vi "Analisi.vi"(6 "Cluster COLORS":cluster{"fore":u32, "back ER":u32, "back":u32}={"fore"=10197915, "back ER"=11796480, "back"=43}, 7 "crea\ntabella scarti":bool, 8 "MCListbox tabella dati":refnum<vi>, 9 "n colonna":i32, 10 "Array index eliminati in":i32[](array[numeric]), 11 "Array":string[](array[string])) -> (2 "Array index eliminati":i32[](array[numeric]))   [LabVIEW 2016]
uses:
  formule.llb/PASSI.ctl
  formule.llb/Global.vi
panel:
  in  "start index (0)":i32
  out "index of element":i32
  out "element":string
  in  "eliminati":i32
  out "Array 2":string[](array[string])
  in  "index":i32
  in  "PASSO":T1
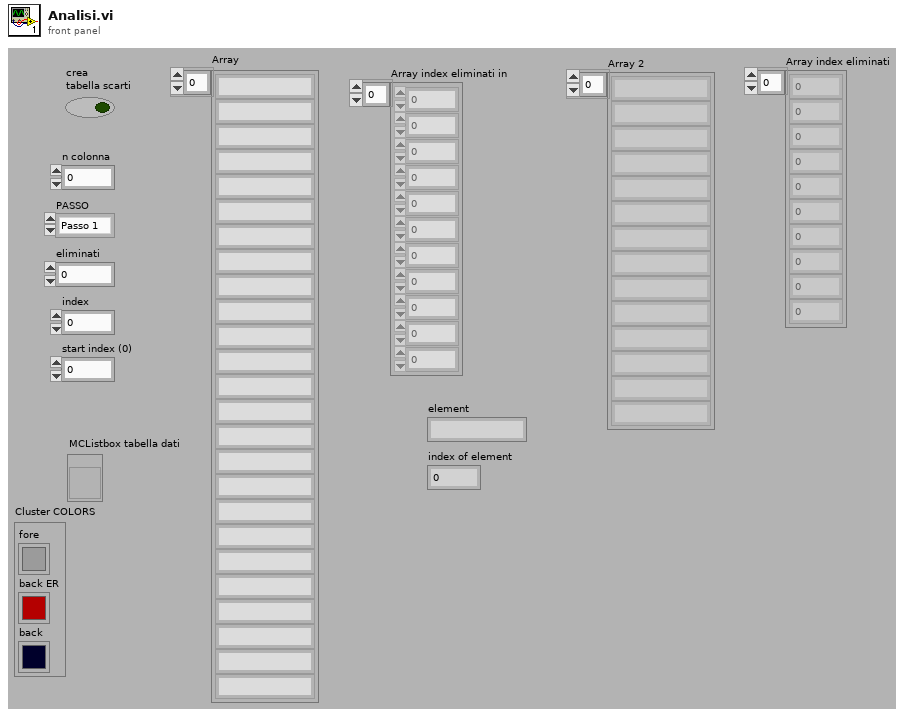
[diagram p1: front panel]
types:
  T1 = typedef "PASSI.ctl" = enum16{"Passo 1", "Passo 2", "Passo 3", "Passo 4", "Passo 5"}
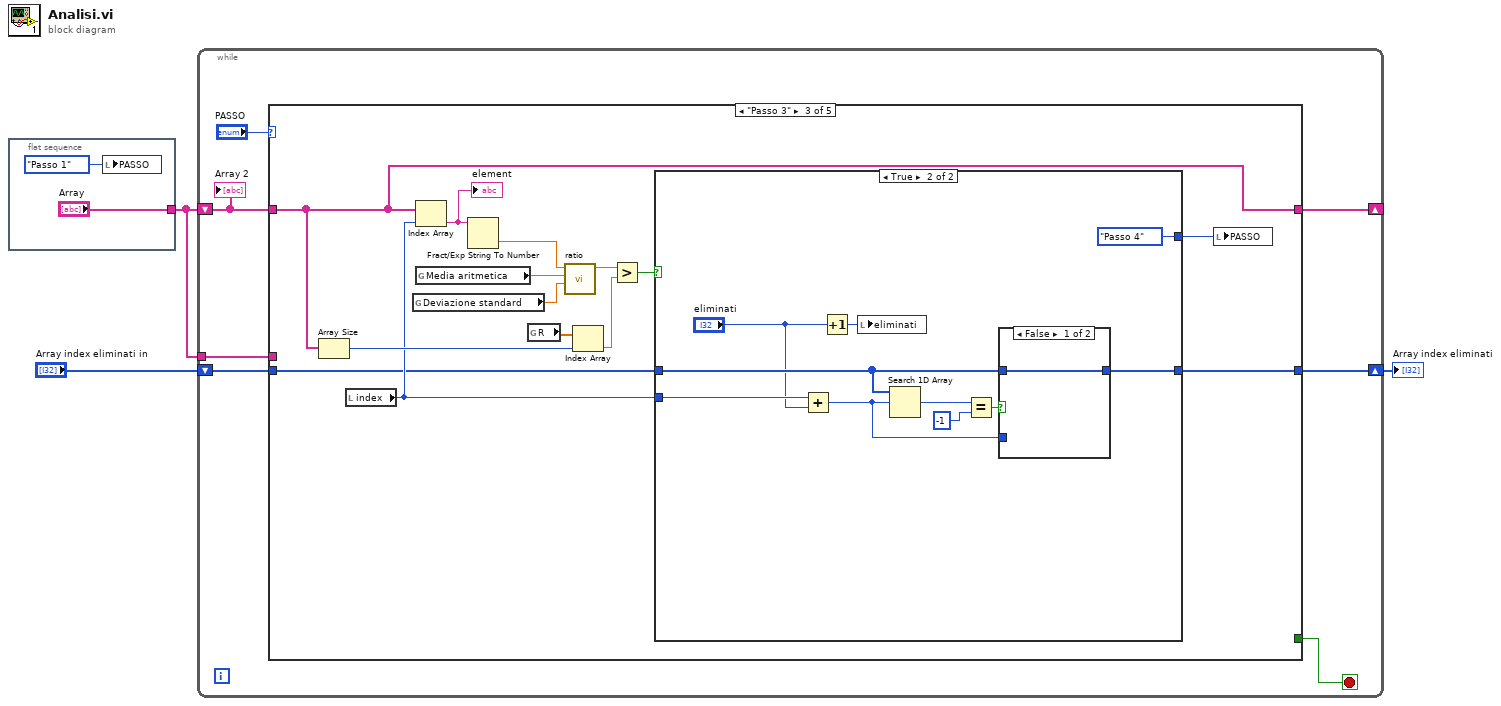
[diagram p0: block diagram]
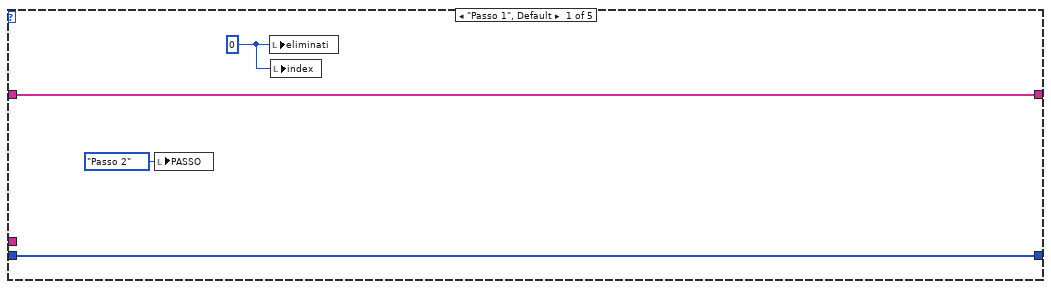
[diagram p2: hidden frame]
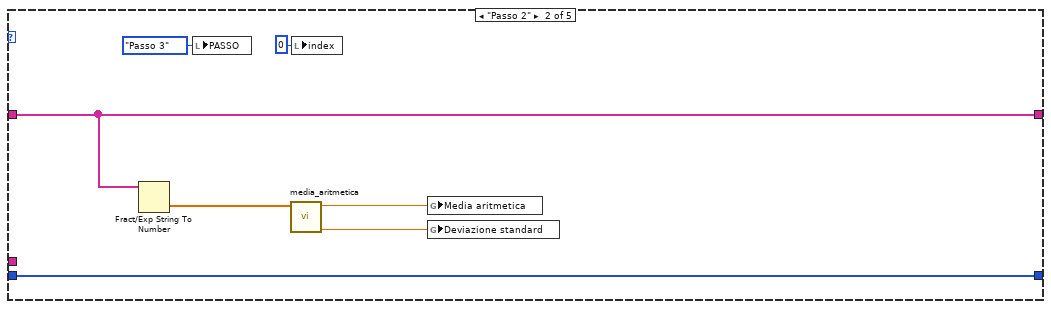
[diagram p3: hidden frame]
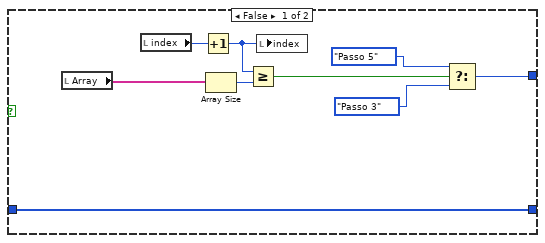
[diagram p4: hidden frame]
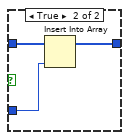
[diagram p5: hidden frame]
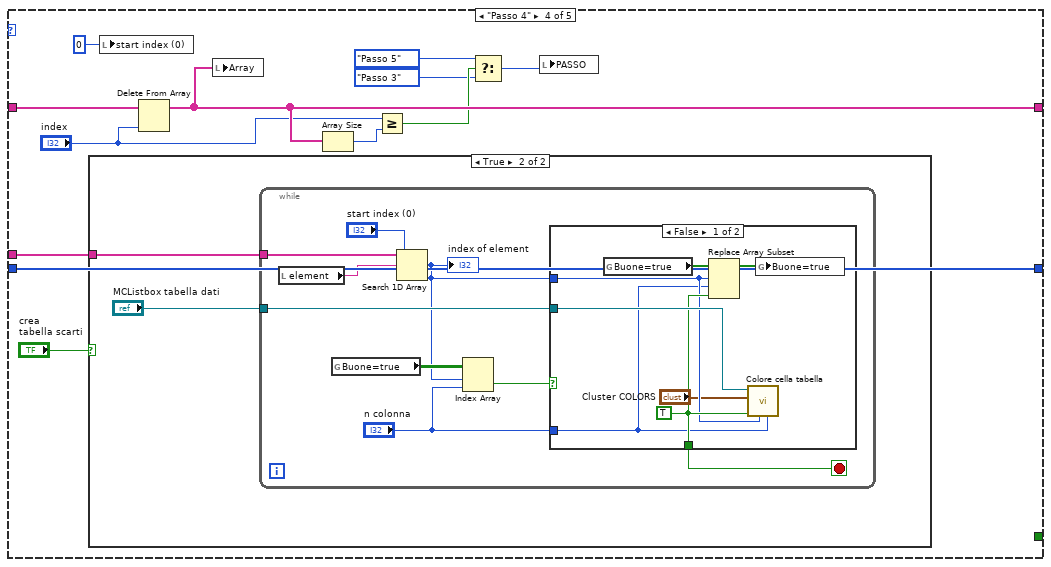
[diagram p6: hidden frame]
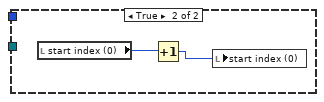
[diagram p8: hidden frame]
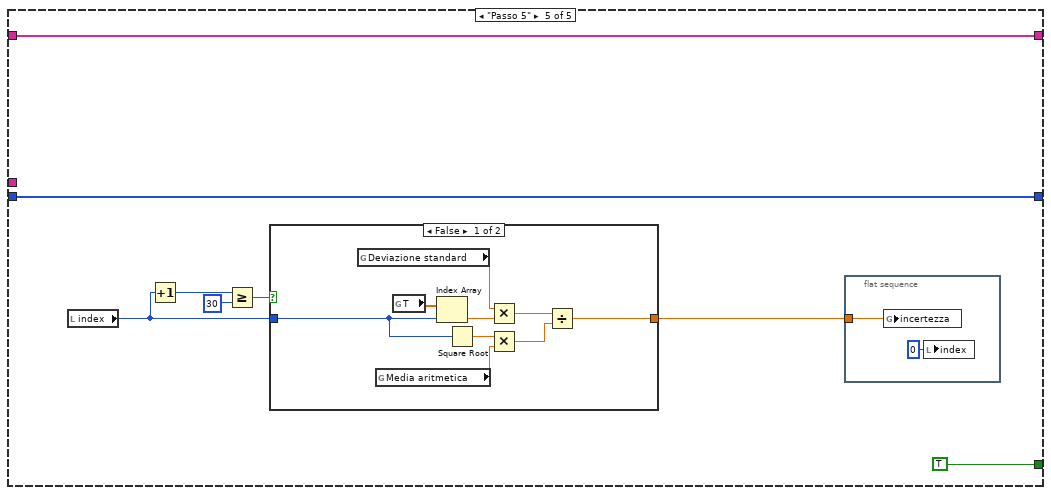
[diagram p9: hidden frame]
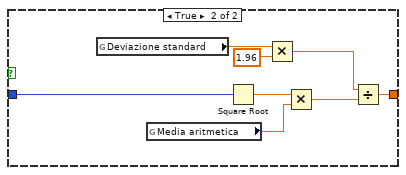
[diagram p10: hidden frame]
diagram:
  n1 = flat-sequence {
    tunnel: ["Array"] -> w1
    frame #0 {
      n2 = local write "PASSO"(PASSI."Passo 1" ("Enum")) -> ()
    }
  }
  n3 = while {
    shift-right: [w9] -> _
    shift-left: w1 -> [w11]
    shift-right: [w8] -> w3
    shift-left: "Array index eliminati in" -> [w7]
    tunnel: w1 -> [w6]
    stop <- w10 stop-if-true
    n4 = case shown="\"Passo 3\"" "PASSO" {
      tunnel: w11 -> [w15 w18 w29 w72 w94]
      tunnel: [_ _ _ _ TRUE ("stop")] -> w10
      tunnel: [w15 w18 w29 w68 w94] -> w9
      tunnel: [w13 w19 w25 w70 w93] -> w8
      tunnel: w7 -> [w13 w19 w24 w70 w93]
      tunnel: w6 -> [_ _ _ w61 _]
      frame "Passo 1", Default {
        w14 = 0 ("index")
        n5 = local write "PASSO"(PASSI."Passo 2" ("Enum")) -> ()
        n6 = local write "eliminati"(w14) -> ()
        n7 = local write "index"(w14) -> ()
      }
      frame "Passo 2" {
        n8 = Fract/Exp String To Number(string=w18) -> (number=w17:dbl[])  [unwired: 4 out]
        n9 = local write "PASSO"(PASSI."Passo 3" ("Enum")) -> ()
        n10 = call "media_aritmetica.vi"("Array"=w17) -> ("Deviazione standard"=w22:dbl, "Media aritmetica"=w23:dbl)  [unwired: 9 out]
        n11 = local write "index"(0 ("index")) -> ()
        n12 = global write "Global.vi" "Media aritmetica"(w23) -> ()
        n13 = global write "Global.vi" "Deviazione standard"(w22) -> ()
      }
      frame "Passo 3" {
        n14 = Array Size(array=w29) -> (size(s)=w28:i32)
        n15 = local read "index"() -> (w27:i32)
        n16 = global read "Global.vi" "Deviazione standard"() -> (w36:dbl)
        n17 = Index Array(array=w29, index=w27) -> (element=w35:string)
        "element" <- w35
        n18 = global read "Global.vi" "Media aritmetica"() -> (w37:dbl)
        n19 = Fract/Exp String To Number(string=w35) -> (number=w34:dbl)  [unwired: 4 out]
        n20 = global read "Global.vi" "R"() -> (w32:dbl[])
        n21 = call "ratio.vi"("Sx"=w36, "Xmedia"=w37, "Xr"=w34) -> ("R"=w33:dbl)  [unwired: 8 out]
        n22 = Index Array(array=w32, index=w28) -> (element=w26:dbl)
        n23 = Greater?(x=w33, y=w26) -> (0:w31:bool)
        n24 = case shown="True" w31 {
          tunnel: [w38 PASSI."Passo 4" ("Enum")] -> w30
          tunnel: w27 -> [_ w49]
          tunnel: [w42 w54] -> w25
          tunnel: w24 -> [w42 w50]
          frame False {
            n25 = local read "Array"() -> (w46:string[])
            n26 = local read "index"() -> (w43:i32)
            n27 = Increment(x=w43) -> (x+1=w45:i32)
            n28 = Array Size(array=w46) -> (size(s)=w44:i32)
            n29 = Greater Or Equal?(x=w45, y=w44) -> (x >= y?=w41:bool)
            n30 = local write "index"(w45) -> ()
            n31 = Select(t=PASSI."Passo 5" ("Enum"), s=w41, f=PASSI."Passo 3" ("Enum")) -> (s? t:f=w38:T1)
          }
          frame True {
            n32 = Add(x=w49, y="eliminati") -> (x+y=w48:i32)
            n33 = Increment(x="eliminati") -> (x+1=w55:i32)
            n34 = local write "eliminati"(w55) -> ()
            n35 = Search 1D Array(1D array=w50, element=w48) -> (index of element=w53:i32)  [unwired: 1 in]
            n36 = Equal?(x=w53, y=-1) -> (x = y?=w51:bool)
            n37 = case shown="False" w51 {
              tunnel: [w57 w60] -> w54
              tunnel: w50 -> [w57 w59]
              tunnel: w48 -> [_ w58]
              frame False {
              }
              frame True {
                n38 = Insert Into Array(array=w59, new element=w58) -> (w60:i32[])  [unwired: 1 in]
              }
            }
          }
        }
        n39 = local write "PASSO"(w30) -> ()
      }
      frame "Passo 4" {
        n40 = case shown="True" "crea\ntabella scarti" {
          tunnel: w61 -> [_ w73]
          frame False {
          }
          frame True {
            n41 = while {
              tunnel: "MCListbox tabella dati" -> [w78]
              tunnel: w73 -> [w75]
              stop <- w79 stop-if-true
              n42 = local read "element"() -> (w83:string)
              n43 = global read "Global.vi" "Buone=true"() -> (w82:bool[][])
              n44 = Search 1D Array(1D array=w75, element=w83, start index (0)="start index (0)") -> (index of element=w77:i32)
              "index of element" <- w77
              n45 = Index Array(array=w82, index (row)=w77, index (col)="n colonna") -> (element=w81:bool)
              n46 = case shown="False" w81 {
                tunnel: "n colonna" -> [w85 _]
                tunnel: w77 -> [w86 _]
                tunnel: [w87 _] -> w79
                tunnel: w78 -> [w88 _]
                frame False {
                  w87 = TRUE ("Boolean")
                  n47 = global read "Global.vi" "Buone=true"() -> (w89:bool[][])
                  n48 = Replace Array Subset(array=w89, new element=w87, index (row)=w86, index (col)=w85) -> (w90:bool[][])
                  n49 = call "Colore cella tabella.vi"("Column"=w85, "Row"=w86, "Vero=rosso"=w87, "Cluster COLORS"="Cluster COLORS", "MCListbox Refnum"=w88) -> ()  [unwired: 2 in, 5 out]
                  n50 = global write "Global.vi" "Buone=true"(w90) -> ()
                }
                frame True {
                  n51 = local read "start index (0)"() -> (w92:i32)
                  n52 = Increment(x=w92) -> (x+1=w91:i32)
                  n53 = local write "start index (0)"(w91) -> ()
                }
              }
            }
          }
        }
        n54 = local write "start index (0)"(0 ("start index (0)")) -> ()
        n55 = Delete From Array(array=w72, index="index") -> (array with subset deleted=w68:string[])  [unwired: 1 in, 1 out]
        n56 = local write "Array"(w68) -> ()
        n57 = Array Size(array=w68) -> (size(s)=w67:i32)
        n58 = Greater Or Equal?(x="index", y=w67) -> (x >= y?=w66:bool)
        n59 = Select(t=PASSI."Passo 5" ("Enum"), s=w66, f=PASSI."Passo 3" ("Enum")) -> (s? t:f=w63:T1)
        n60 = local write "PASSO"(w63) -> ()
      }
      frame "Passo 5" {
        n61 = local read "index"() -> (w97:i32)
        n62 = Increment(x=w97) -> (x+1=w98:i32)
        n63 = Greater Or Equal?(x=w98, y=30) -> (x >= y?=w99:bool)
        n64 = case shown="False" w99 {
          tunnel: w97 -> [w108 w114]
          tunnel: [w103 w112] -> w96
          frame False {
            n65 = global read "Global.vi" "Deviazione standard"() -> (w107:dbl)
            n66 = global read "Global.vi" "Media aritmetica"() -> (w110:dbl)
            n67 = global read "Global.vi" "T"() -> (w106:dbl[])
            n68 = Index Array(array=w106, index=w108) -> (element=w105:dbl)
            n69 = Square Root(x=w108) -> (sqrt(x)=w111:dbl)
            n70 = Multiply(x=w107, y=w105) -> (x*y=w104:dbl)
            n71 = Multiply(x=w111, y=w110) -> (x*y=w109:dbl)
            n72 = Divide(x=w104, y=w109) -> (x/y=w103:dbl)
          }
          frame True {
            n73 = global read "Global.vi" "Deviazione standard"() -> (w119:dbl)
            n74 = global read "Global.vi" "Media aritmetica"() -> (w115:dbl)
            n75 = Square Root(x=w114) -> (sqrt(x)=w116:dbl)
            n76 = Multiply(x=w119, y=1.96) -> (x*y=w117:dbl)
            n77 = Multiply(x=w116, y=w115) -> (x*y=w113:dbl)
            n78 = Divide(x=w117, y=w113) -> (x/y=w112:dbl)
          }
        }
        n79 = flat-sequence {
          tunnel: w96 -> [w102]
          frame #0 {
            n80 = global write "Global.vi" "incertezza"(w102) -> ()
            n81 = local write "index"(0 ("index")) -> ()
          }
        }
      }
    }
    "Array 2" <- w11
  }
  "Array index eliminati" <- w3
